vi "QuickDrop Enable Subdiagram.vi"(6 "Variant in":variant, 7 "Shift Pressed?":bool, 8 "error in (no error)":errorcluster, 10 "QD Combo Box Ref":refnum<vi>, 11 "QD Launch VI Ref":refnum<vi>) -> (0 "error out":errorcluster, 4 "Variant out":variant)   [LabVIEW 2013]
doc: "Enables the visible Diagram Disable Frame\nHolding Shift removes the Structure entirely\n\nDefault Shortcut - [E]"
panel:
  in  "Shift Undo Name":string="Remove Diagram Disable Structure"
  in  "Undo Name":string="Enable Visible Diagram Disable Subdiagram"
  # "Do not change the connector pane of this VI.\n\nSee the block diagram for directions on how to use this template."
  # "Specify the name of the Undo transaction"
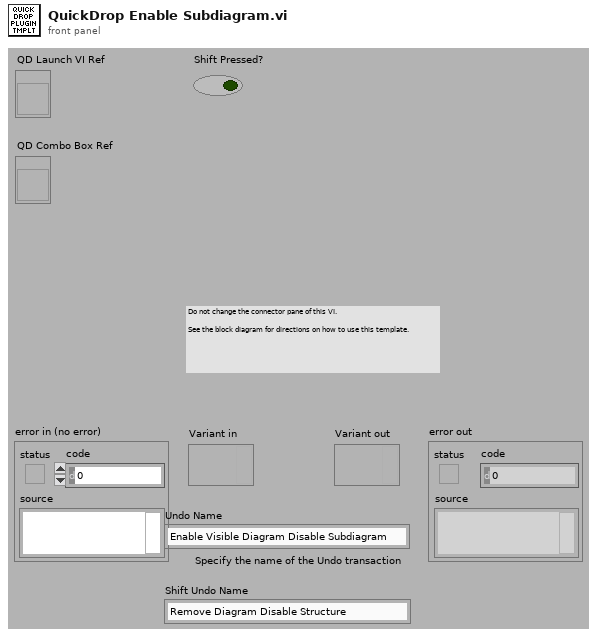
[diagram p1: front panel]
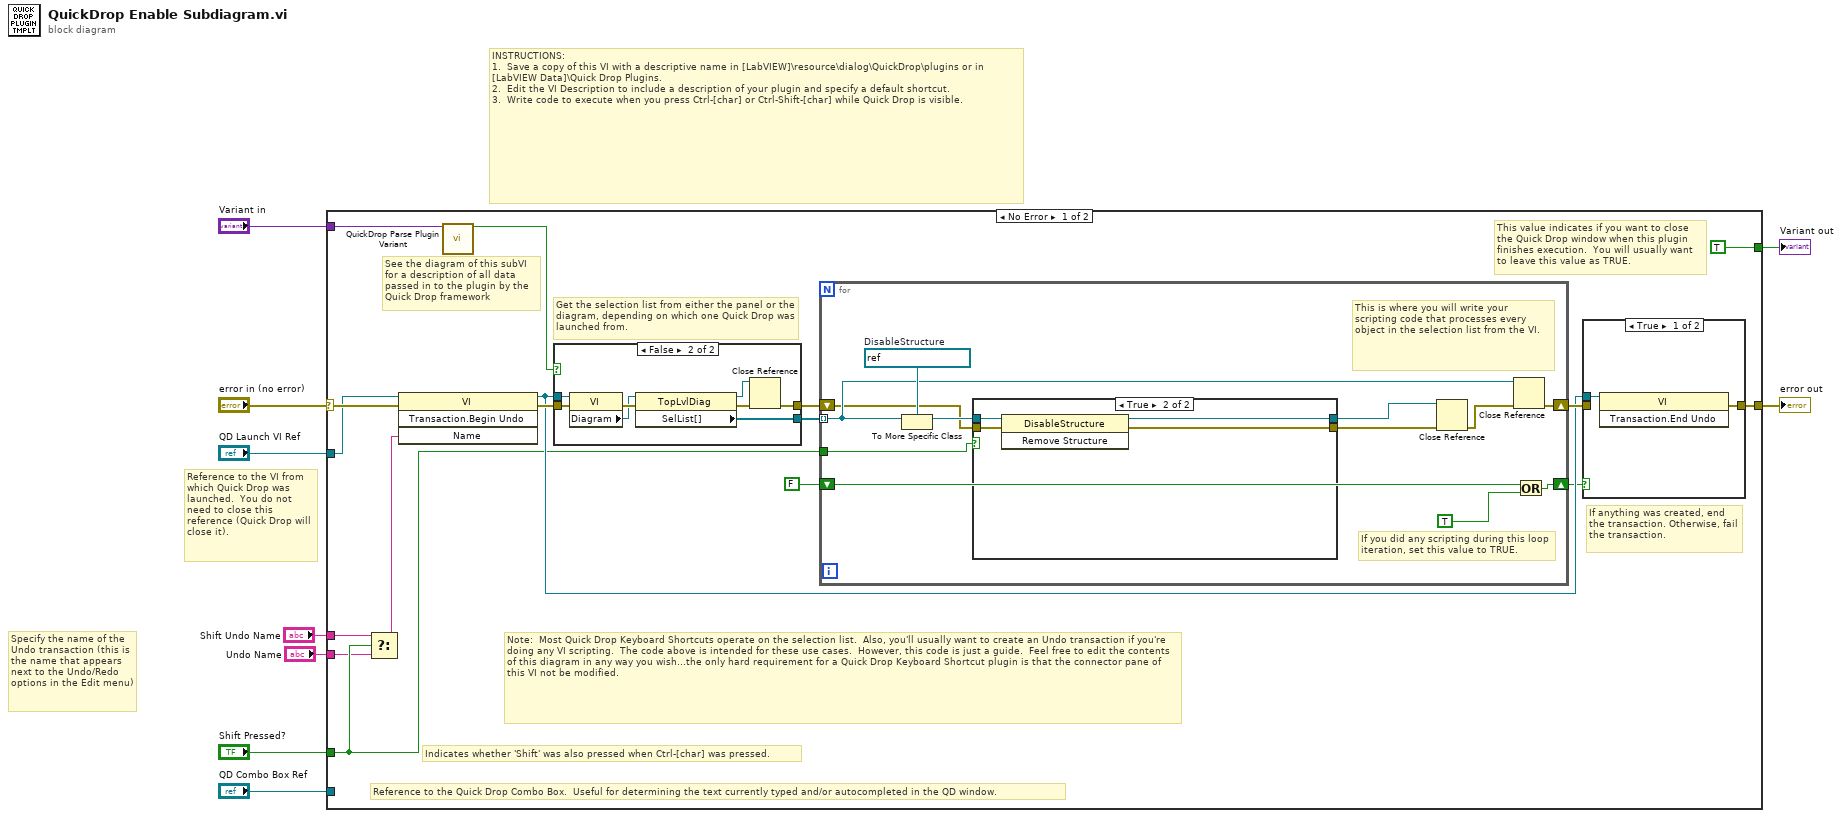
[diagram p0: block diagram]
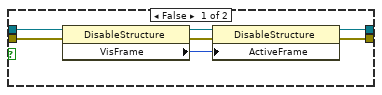
[diagram p2: hidden frame]
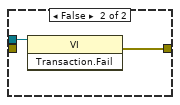
[diagram p3: hidden frame]
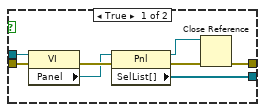
[diagram p4: hidden frame]
diagram:
  # "Specify the name of the Undo transaction (this is the name that appears next to the Undo/Redo options in the Edit menu)"
  # "Reference to the VI from which Quick Drop was launched.  You do not need to close this reference (Quick Drop will close it)."
  # "INSTRUCTIONS:\n1.  Save a copy of this VI with a descriptive name in [LabVIEW]\\resource\\dialog\\QuickDrop\\plugins or in [LabVIEW Data]\\Quick Drop Plugins.\n2.  Edit the VI Description to include a description of your plugin and specify a default shortcut. \n3.  Write code to execute when you press Ctrl-[char] or Ctrl-Shift-[char] while Quick Drop is visible."
  n1 = case shown="No Error" "error in (no error)" {
    selector: "error in (no error)" -> [w25 w70]
    tunnel: [w20 w70] -> w8
    tunnel: "QD Launch VI Ref" -> [w24 _]
    tunnel: "Shift Pressed?" -> [w13 _]
    tunnel: "QD Combo Box Ref" -> [_ _]
    tunnel: "Variant in" -> [w26 _]
    tunnel: "Undo Name" -> [w12 _]
    tunnel: [TRUE _] -> w2
    tunnel: "Shift Undo Name" -> [w11 _]
    frame No Error {
      # "Note:  Most Quick Drop Keyboard Shortcuts operate on the selection list.  Also, you'll usually want to create an Undo transaction if you're doing any VI scripting.  The code above is intended for these use cases.  However, this code is just a guide.  Feel free to edit the contents of this diagram in any way you wish...the only hard requirement for a Quick Drop Keyboard Shortcut plugin is that the connector pane of this VI not be modified."
      # "Get the selection list from either the panel or the diagram, depending on which one Quick Drop was launched from."
      # "If anything was created, end the transaction. Otherwise, fail the transaction."
      # "This value indicates if you want to close the Quick Drop window when this plugin finishes execution.  You will usually want to leave this value as TRUE."
      # "See the diagram of this subVI for a description of all data passed in to the plugin by the Quick Drop framework"
      # "Reference to the Quick Drop Combo Box.  Useful for determining the text currently typed and/or autocompleted in the QD window."
      # "Indicates whether 'Shift' was also pressed when Ctrl-[char] was pressed."
      n2 = Select(t=w11, s=w13, f=w12) -> (s? t:f=w10:string)
      n3 = invoke class="VI" method="Transaction.Begin Undo"(reference=w24, error in=w25, "Name"=w10) -> (reference out=w17:refnum<vi>, error out=w21:errorcluster)  [unwired: 1 in, 2 out]
      n4 = call <vilib>:"QuickDrop Parse Plugin Variant.vi"("QDKS Variant in"=w26) -> ("QD Launch VI Panel?"=w22:bool)  [unwired: 12 in, 2 out]
      n5 = case shown="False" w22 {
        tunnel: w21 -> [w61 w69]
        tunnel: w17 -> [w60 w68]
        tunnel: [w55 w63] -> w19
        tunnel: [w54 w62] -> w14
        frame True {
          n6 = property class="VI"(reference=w60, error in=w61) -> (error out=w59:errorcluster, "Panel"=w58:refnum<vi>)  [unwired: 1 out]
          n7 = property class="Pnl"(reference=w58, error in=w59) -> (reference out=w56:refnum<vi>, error out=w57:errorcluster, "SelList[]"=w54:refnum<vi>[])
          n8 = Close Reference(reference=w56, error in (no error)=w57) -> (error out=w55:errorcluster)
        }
        frame False {
          n9 = property class="VI"(reference=w68, error in=w69) -> (error out=w67:errorcluster, "Diagram"=w66:refnum<vi>)  [unwired: 1 out]
          n10 = property class="TopLvlDiag"(reference=w66, error in=w67) -> (reference out=w64:refnum<vi>, error out=w65:errorcluster, "SelList[]"=w62:refnum<vi>[])
          n11 = Close Reference(reference=w64, error in (no error)=w65) -> (error out=w63:errorcluster)
        }
      }
      n12 = for {
        shift-right: [w35] -> w18
        shift-left: w19 -> [w31]
        shift-right: [w37] -> w15
        shift-left: FALSE -> [w38]
        tunnel: w14 -> [w33] mode=indexing
        tunnel: w13 -> [w30]
        w34 = refnum<vi> refnum  # DisableStructure
        # "This is where you will write your scripting code that processes every object in the selection list from the VI."
        # "If you did any scripting during this loop iteration, set this value to TRUE."
        n13 = To More Specific Class(target class=w34, reference=w33) -> (specific class reference=w32:refnum<vi>)  [unwired: 1 in, 1 out]
        n14 = case shown="True" w30 {
          tunnel: w32 -> [w45 w49]
          tunnel: w31 -> [w44 w48]
          tunnel: [w41 w47] -> w29
          tunnel: [w39 w46] -> w27
          frame False {
            n15 = property class="DisableStructure"(reference=w45, error in=w44) -> (reference out=w43:refnum<vi>, error out=w42:errorcluster, "VisFrame"=w40:u32)
            n16 = property class="DisableStructure"(reference=w43, error in=w42, "ActiveFrame"=w40) -> (reference out=w39:refnum<vi>, error out=w41:errorcluster)
          }
          frame True {
            n17 = invoke class="DisableStructure" method="Remove Structure"(reference=w49, error in=w48) -> (reference out=w46:refnum<vi>, error out=w47:errorcluster)  [unwired: 1 in, 1 out]
          }
        }
        n18 = Close Reference(reference=w27, error in (no error)=w29) -> (error out=w28:errorcluster)
        n19 = Close Reference(reference=w33, error in (no error)=w28) -> (error out=w35:errorcluster)
        n20 = Or(x=w38, y=TRUE ("x")) -> (x .or. y?=w37:bool)
      }
      n21 = case shown="True" w15 {
        tunnel: w17 -> [w50 w52]
        tunnel: [w51 w53] -> w20
        tunnel: w18 -> [_ _]
        frame True {
          n22 = invoke class="VI" method="Transaction.End Undo"(reference=w50) -> (error out=w51:errorcluster)  [unwired: 2 in, 2 out]
        }
        frame False {
          n23 = invoke class="VI" method="Transaction.Fail"(reference=w52) -> (error out=w53:errorcluster)  [unwired: 2 in, 2 out]
        }
      }
    }
    frame Error {
    }
  }
  "error out" <- w8
  "Variant out" <- w2
